vi "fbeta.vi"(9 "Ankle Angle":dbl, 10 "Constants and System Parameters":T1) -> (2 "fbeta":dbl)   [LabVIEW 2018]
uses:
  Constants and System Parameters.ctl
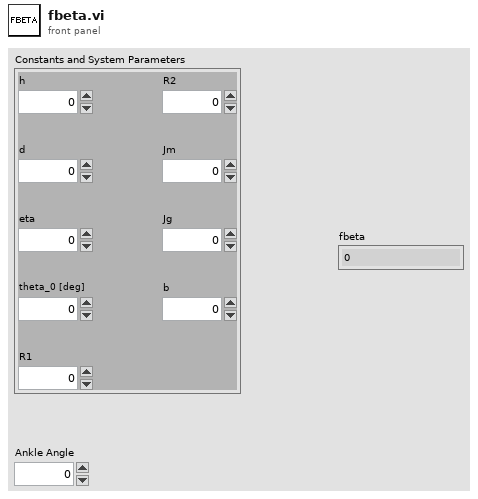
[diagram p1: front panel]
types:
  T1 = typedef "Constants and System Parameters.ctl" = cluster{"h":dbl, "d":dbl, "eta":dbl, "theta_0 [deg]":dbl, "R1":dbl, "R2":dbl, "Jm":dbl, "Jg":dbl, "b":dbl}
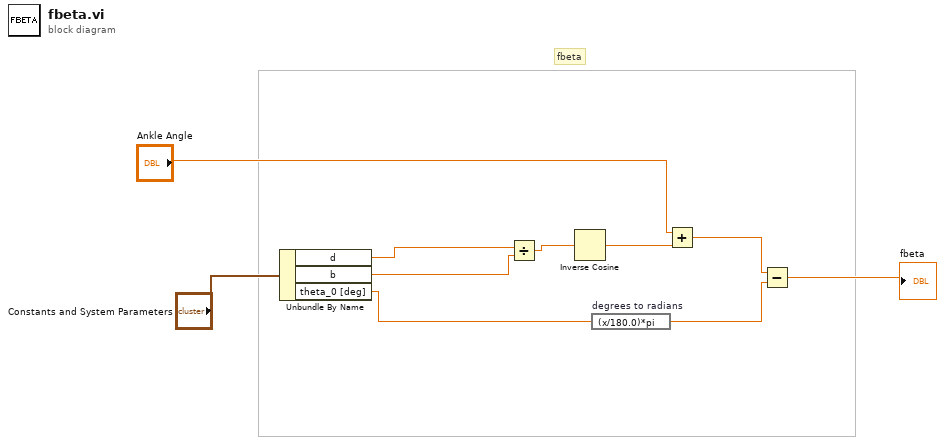
[diagram p0: block diagram]
diagram:
  # "fbeta"
  n1 = Unbundle By Name("Constants and System Parameters") -> ("d"=w6:dbl, "b"=w2:dbl, "theta_0 [deg]"=w1:dbl)
  n2 = Divide(x=w6, y=w2) -> (x/y=w10:dbl)
  n3 = Inverse Cosine(1:w10) -> (0:w9:dbl)
  n4 = expression code="(x/180.0)*pi" "degrees to radians"(w1) -> (w7:dbl)
  n5 = Add(x="Ankle Angle", y=w9) -> (x+y=w8:dbl)
  n6 = Subtract(x=w8, y=w7) -> (x-y=→"fbeta":dbl)
